vi "Disconnect Channels (Multiple).vi"(8 "error in (no error)":errorcluster, 10 "disconnection list":string, 11 "session in":T1) -> (0 "error out":errorcluster, 3 "session out":T1)   [LabVIEW 2020, in "SLSC Switch.lvlib"]
doc: "Breaks the connections between channels specified in <B>disconnection list</B>. If no connections exist between channels, NI-SLSC Switch returns an error. In the event of an error, the VI stops at the point in the list where the error occurred."
uses:
  <vilib>/SLSC_Switch/SLSC Switch.lvlib
  nislscsl.dll
  <vilib>/userdefined/High Color/SLSC_Switch/nislscslSession.ctl
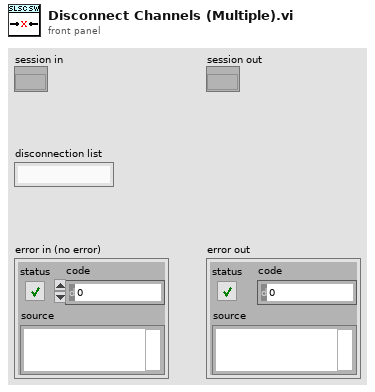
[diagram p1: front panel]
types:
  T1 = typedef "nislscslSession.ctl" = refnum<k20>
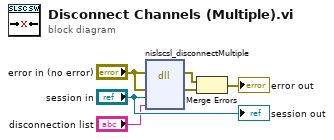
[diagram p0: block diagram]
diagram:
  n1 = dll-call lib="nislscsl.*" fn="nislscsl_disconnectMultiple"(error in="error in (no error)", "errorCluster"="error in (no error)", "sessionHandle"="session in", "disconnectionList"="disconnection list") -> (error out=w6:errorcluster, "errorCluster"=w5:errorcluster)  [unwired: 5 in, 1 out]
  n2 = Merge Errors(w6, w5) -> (→"error out":errorcluster)
  "session out" <- "session in"
